vi "RTS Equipment Send TCP Data.vi"(7 "RTS Config Setup Input":T3, 8 "Error In":errorcluster, 9 "TDMS Data Save":T1, 10 "Data":T12, 11 "Send Data":string[][](array[string])) -> (0 "Error Out":errorcluster, 1 "# of Connections":i32, 2 "Data Out":T12, 3 "RTS Config Setup Output":T3, 4 "Custom Commands":string[](array[string]), 5 "TDMS Data Save Output":T1, 6 "Read Door CMD":string)   [LabVIEW 2016]
uses:
  Type Definitions/RTS TCP Multiple Connections Data.ctl
  Type Definitions/RTS Configuration Setup.ctl
  Type Definitions/RTS Wago Config.ctl
  Type Definitions/RTS APLUS Config.ctl
  Type Definitions/RTS Yokogawa MX Config.ctl
  Type Definitions/RTS Replay Server Control.ctl
  Type Definitions/RTS Server Configuration.ctl
  Type Definitions/RTS Station Settions TCP Comms.ctl
  Type Definitions/RTS Chamber Save Status.ctl
  Type Definitions/RTS Test Pattern.ctl
  Type Definitions/RTS TDMS Filename Locations.ctl
  Type Definitions/RTS Save References.ctl
panel:
  out "TCP Command":string
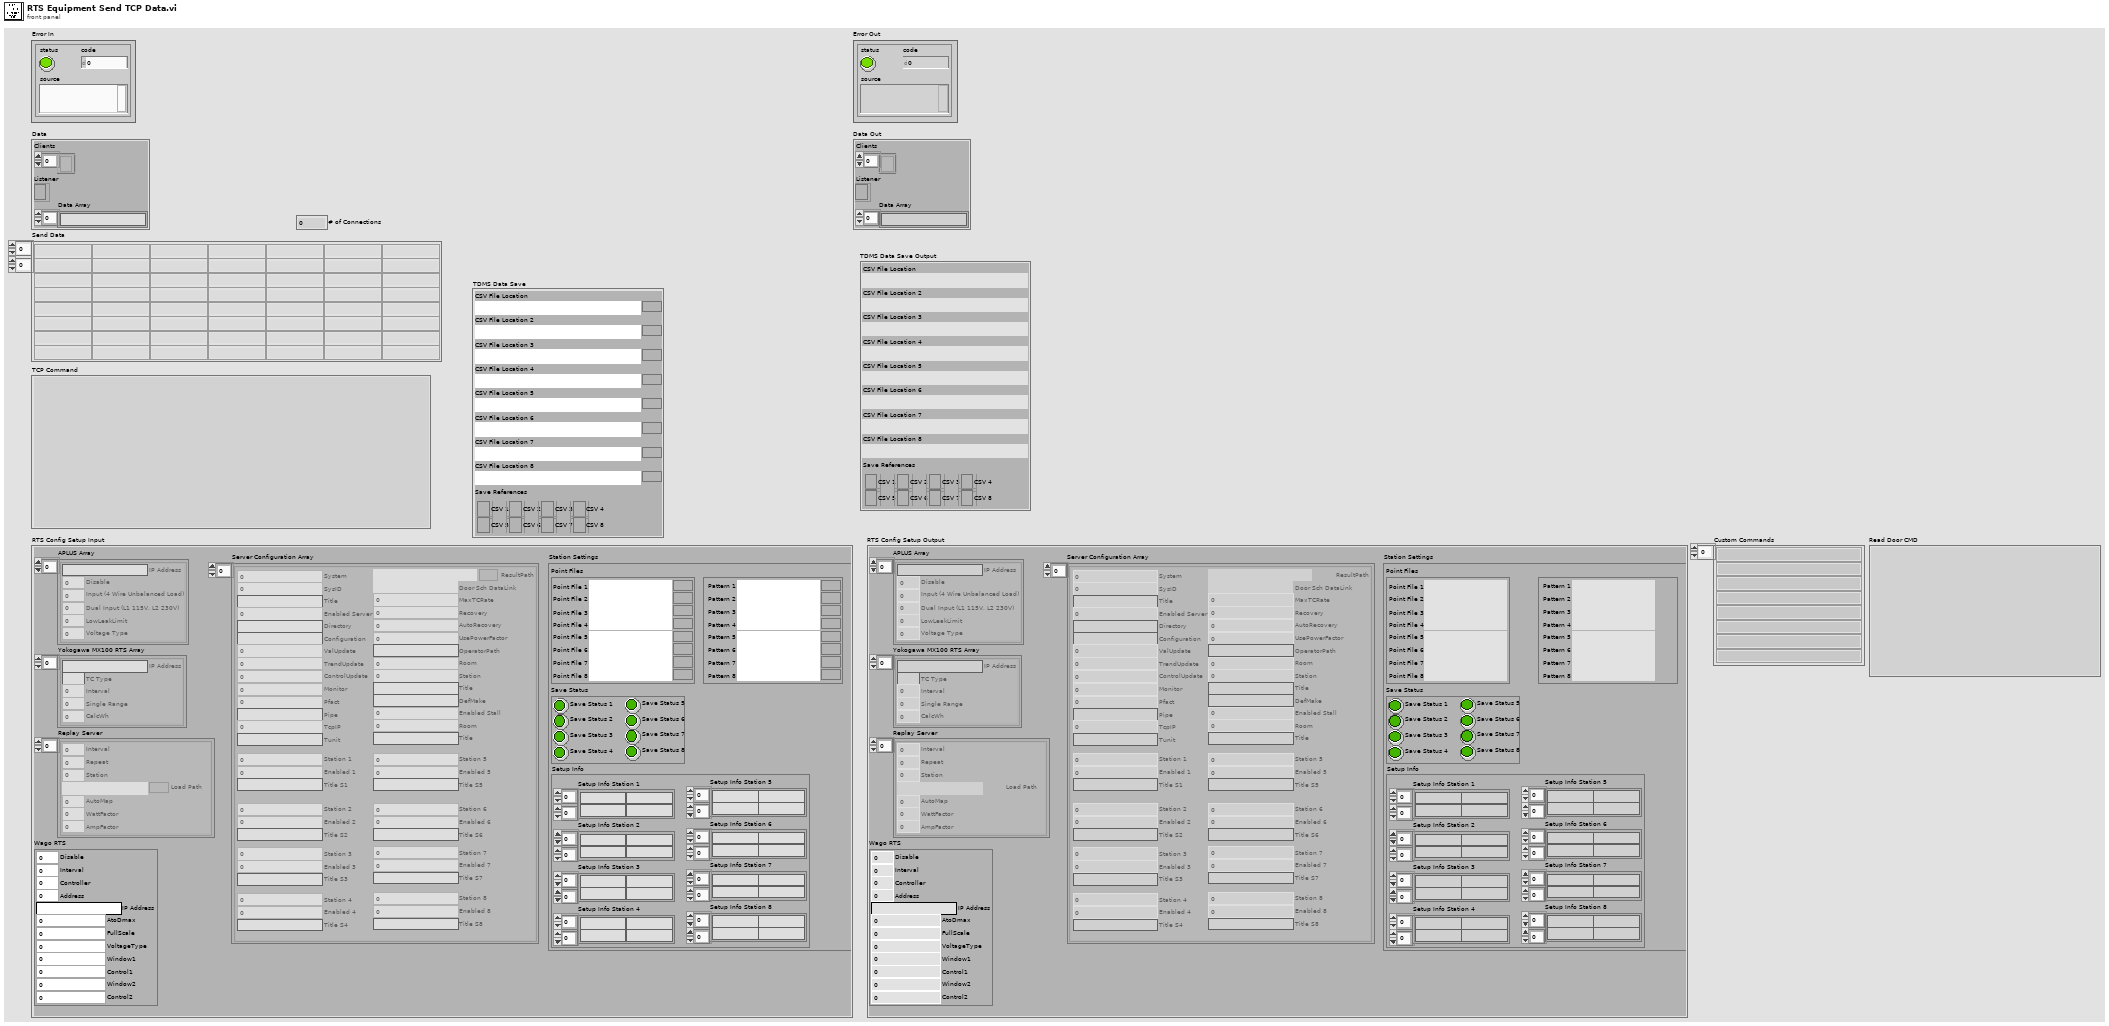
[diagram p1: front panel]
types:
  T1 = typedef "RTS TDMS Filename Locations.ctl" = cluster{"CSV File Location":path, "CSV File Location 2":path, "CSV File Location 3":path, "CSV File Location 4":path, "CSV File Location 5":path, "CSV File Location 6":path, "CSV File Location 7":path, "CSV File Location 8":path, "Save References":T2}
  T2 = typedef "RTS Save References.ctl" = cluster{"CSV 1":refnum<file>, "CSV 2":refnum<file>, "CSV 3":refnum<file>, "CSV 4":refnum<file>, "CSV 5":refnum<file>, "CSV 6":refnum<file>, "CSV 7":refnum<file>, "CSV 8":refnum<file>}
  T3 = typedef "RTS Configuration Setup.ctl" = cluster{"Wago RTS":T4, "APLUS Array":T5[], "Yokogawa MX100 RTS Array":T6[], "Replay Server":T7[], "Server Configuration Array":T8[], "Station Settings":T9}
  T4 = typedef "RTS Wago Config.ctl" = cluster{"Disable":u16, "Interval":u16, "Controller":u16, "Address":u16, "IP Address":string, "AtoDmax":u16, "FullScale":u16, "VoltageType":u16, "Window1":u16, "Control1":u16, "Window2":u16, "Control2":u16}
  T5 = typedef "RTS APLUS Config.ctl" = cluster{"Disable":u16, "IP Address":string, "Input (4 Wire Unbalanced Load)":u16, "Dual Input (L1 115V, L2 230V)":u16, "LowLeakLimit":dbl, "Voltage Type":u16}
  T6 = typedef "RTS Yokogawa MX Config.ctl" = cluster{"IP Address":string, "TC Type":string, "Interval":u16, "Single Range":u16, "CalcWh":u16}
  T7 = typedef "RTS Replay Server Control.ctl" = cluster{"Interval":i16, "Repeat":u16, "Station":u16, "Load Path":path, "AutoMap":u16, "WattFactor":dbl, "AmpFactor":dbl}
  T8 = typedef "RTS Server Configuration.ctl" = cluster{"System":u16, "SysID":u16, "Title":string, "Enabled Server":u16, "Directory":string, "Configuration":string, "ValUpdate":u16, "TrendUpdate":u16, "ControlUpdate":u16, "Monitor":u16, "Pfact":u16, "Pipe":string, "TcpIP":u16, "Tunit":string, "ResultPath":path, "Door Sch DataLink":path, "MaxTCRate":u16, "Recovery":u16, "AutoRecovery":u16, "UsePowerFactor":u16, "OperatorPath":string, "Room":u16, "Station":u16, "Title":string, "DefMake":string, "Enabled Stall":u16, "Room":u16, "Title":string, "Station 1":u16, "Enabled 1":u16, "Station 2":u16, "Enabled 2":u16, "Station 3":u16, "Enabled 3":u16, "Station 4":u16, "Enabled 4":u16, "Station 5":u16, "Enabled 5":u16, "Station 6":u16, "Enabled 6":u16, "Station 7":u16, "Enabled 7":u16, "Station 8":u16, "Enabled 8":u16, "Title S1":string, "Title S2":string, "Title S3":string, "Title S5":string, "Title S6":string, "Title S7":string, "Title S8":string, "Title S4":string}
  T9 = typedef "RTS Station Settions TCP Comms.ctl" = cluster{"Point Files":cluster{"Point File 1":path, "Point File 2":path, "Point File 3":path, "Point File 4":path, "Point File 5":path, "Point File 6":path, "Point File 7":path, "Point File 8":path}, "Save Status":T10, "Setup Info":cluster{"Setup Info Station 1":string[][], "Setup Info Station 2":string[][], "Setup Info Station 3":string[][], "Setup Info Station 4":string[][], "Setup Info Station 5":string[][], "Setup Info Station 6":string[][], "Setup Info Station 7":string[][], "Setup Info Station 8":string[][]}, "Chamber Test Pattern":T11}
  T10 = typedef "RTS Chamber Save Status.ctl" = cluster{"Save Status 1":bool, "Save Status 2":bool, "Save Status 3":bool, "Save Status 4":bool, "Save Status 5":bool, "Save Status 6":bool, "Save Status 7":bool, "Save Status 8":bool}
  T11 = typedef "RTS Test Pattern.ctl" = cluster{" Pattern 1":path, "Pattern 2":path, "Pattern 3":path, "Pattern 4":path, "Pattern 5":path, "Pattern 6":path, "Pattern 7":path, "Pattern 8":path}
  T12 = typedef "RTS TCP Multiple Connections Data.ctl" = cluster{"Clients":refnum<k5>[], "Listener":refnum<k5>, "Data Array":string[]}
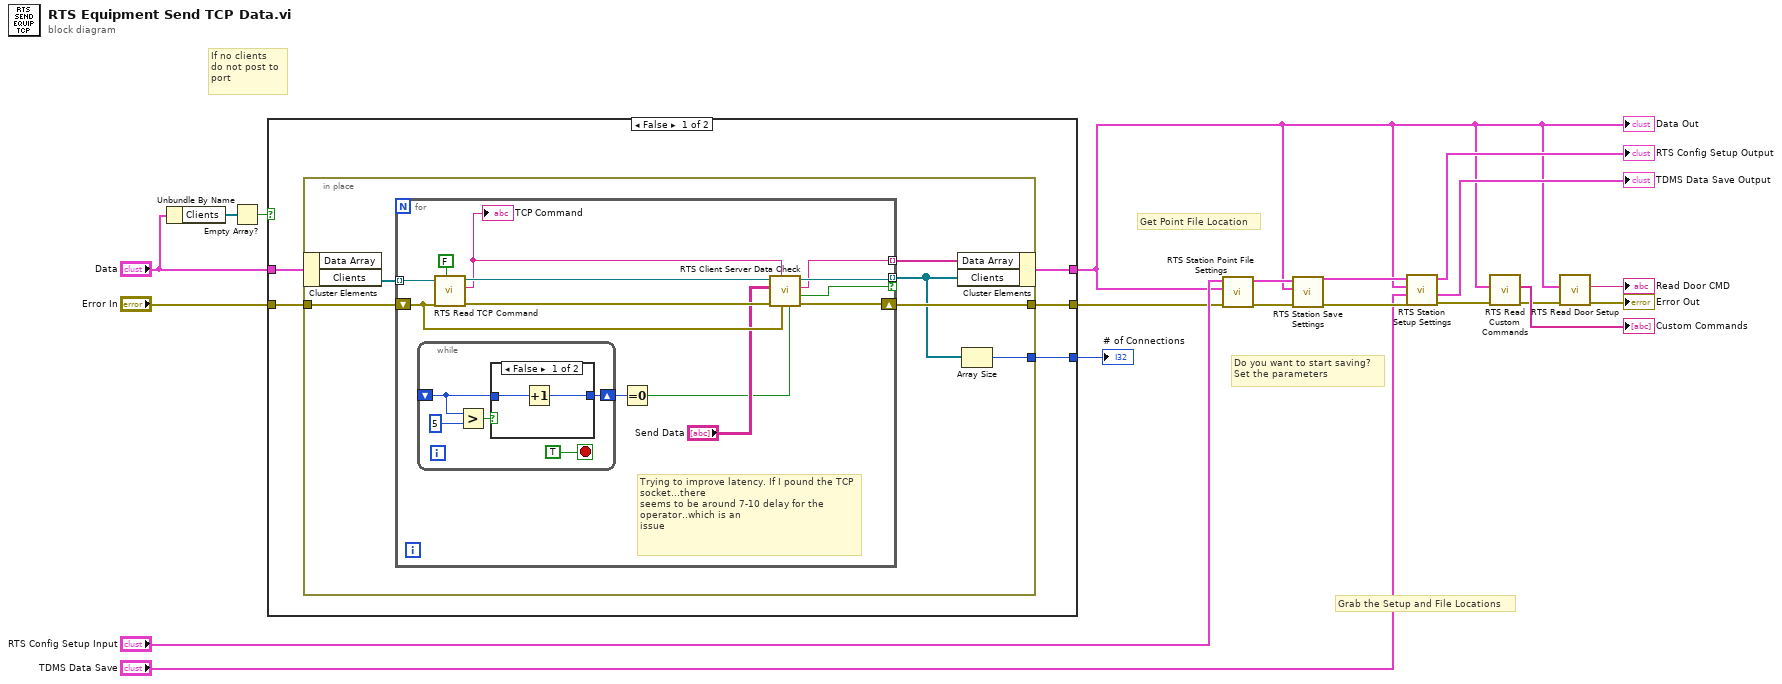
[diagram p0: block diagram]
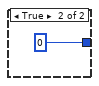
[diagram p2: hidden frame]
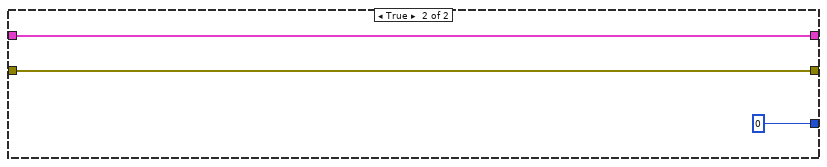
[diagram p3: hidden frame]
diagram:
  # "Get Point File Location"
  # "Do you want to start saving?\nSet the parameters"
  # "Grab the Setup and File Locations"
  # "If no clients\ndo not post to\nport"
  n1 = Unbundle By Name("Data") -> ("Clients"=w18:refnum<k5>[])
  n2 = Empty Array?(array=w18) -> (empty?=w16:bool)
  n3 = case shown="False" w16 {
    tunnel: [w25 0] -> w20
    tunnel: "Data" -> [w24 w55]
    tunnel: "Error In" -> [w23 w54]
    tunnel: [w22 w54] -> w14
    tunnel: [w21 w55] -> w3
    frame False {
      n4 = in-place {
        in-place-border: w23 -> [w31]
        in-place-border: [w30] -> w22
        in-place-border: [w27] -> w25
        n5 = in-place-cluster #1(w24) -> ("Clients"=w29:refnum<k5>[])  [unwired: 1 out]
        n6 = for {
          tunnel: w29 -> [w44] mode=indexing
          shift-right: [w40] -> w30
          shift-left: w31 -> [w36]
          tunnel: [w39] -> w28 mode=indexing if=w41
          tunnel: [w38] -> w26 mode=indexing
          # "Trying to improve latency. If I pound the TCP socket...there\nseems to be around 7-10 delay for the operator..which is an\nissue"
          n7 = while {
            shift-right: [w45] -> w33
            shift-left: _ -> [w46]
            stop <- TRUE stop-if-true
            n8 = Greater?(x=w46, y=u8 5) -> (0:w48:bool)
            n9 = case shown="False" w48 {
              tunnel: w46 -> [w51 _]
              tunnel: [w50 u8 0] -> w45
              frame False {
                n10 = Increment(x=w51) -> (x+1=w50:u8)
              }
              frame True {
              }
            }
          }
          n11 = call "RTS Read TCP Command.vi"("Client Side?"=FALSE, "error in (no error)"=w36, "TCP Network Connection in"=w44) -> ("error out"=w43:errorcluster, "TCP Command"=w34:string, "TCP Network Connection out"=w42:refnum<k5>)  [unwired: 5 in, 1 out]
          "TCP Command" <- w34
          n12 = Equal To 0?(x=w33) -> (x = 0?=w32:bool)
          n13 = call "RTS Client Server Data Check.vi"("Skip Data Send"=w32, "error in (no error)"=w36, "TCP Command"=w34, "error IO"=w43, "Send Data"="Send Data", "TCP Network Connection in"=w42) -> ("error out"=w40:errorcluster, "Boolean"=w41:bool, "data out"=w38:string, "TCP Network Connection out"=w39:refnum<k5>)  [unwired: 2 in]
        }
        n14 = in-place-cluster #1("Data Array"=w26, "Clients"=w28) -> (w21:T12)
        n15 = Array Size(array=w28) -> (size(s)=w27:i32)
      }
    }
    frame True {
    }
  }
  "# of Connections" <- w20
  "Data Out" <- w3
  n16 = call "RTS Station Point File Settings.vi"("Error In"=w14, "Data"=w3, "RTS Config Setup Input"="RTS Config Setup Input") -> ("Error Out"=w13:errorcluster, "RTS Config Setup Output"=w12:T3)  [unwired: 7 in]
  n17 = call "RTS Station Save Settings.vi"("Error In"=w13, "Data"=w3, "RTS Config Setup Input"=w12) -> ("Error Out"=w11:errorcluster, "RTS Config Setup Output"=w10:T3)  [unwired: 7 in]
  n18 = call "RTS Station Setup Settings.vi"("Error In"=w11, "TDMS Data Save Input"="TDMS Data Save", "Data"=w3, "RTS Config Setup Input"=w10) -> ("Error Out"=w6:errorcluster, "TDMS Data Save Output"=→"TDMS Data Save Output":T1, "RTS Config Setup Output"=→"RTS Config Setup Output":T3)  [unwired: 5 in]
  n19 = call "RTS Read Custom Commands.vi"("Error In"=w6, "Data Out"=w3) -> ("Error Out"=w4:errorcluster, "Custom Commands"=→"Custom Commands":string[])  [unwired: 8 in]
  n20 = call "RTS Read Door Setup.vi"("Error In"=w4, "Data Out"=w3) -> ("Error Out"=→"Error Out":errorcluster, "Read Door CMD"=→"Read Door CMD":string)  [unwired: 8 in]
